vi "E517_Simple_Test.vi"(0 "System no.":i32=1 min=1 step=1, 5 "error in":errorcluster, 6 "Interface":u16(ring) items=["RS232", "GPIB", "TCP/IP", "USB"], 7 "Timeout":u32=5000, 8 "RS232 settings":cluster{"Portnumber":i32, "Baudrate":u16}={"Portnumber"=0, "Baudrate"=5} {"Portnumber" items=["COM1", "COM2", "COM3", "COM4", "COM5", "COM6", "COM7", "COM8", "COM9", "COM10", "COM11", "COM12", "COM13", "COM14", "COM15", "COM16", "COM17", "COM18", "COM19", "COM20", "COM21", "COM22", "COM23", "COM24", "COM25", "COM26", "COM27", "COM28", "COM29", "COM30"]; "Baudrate" items=["9600", "14400", "19200", "38400", "57600", "115200"]}, 9 "GPIB settings":cluster{"Bus":i32, "Address":i32}={"Bus"=0, "Address"=4}, 10 "TCP/IP settings":T1={"Host address/name"="localhost", "Port"=50000, "Board"=0, "TCP/IP Search?"=TRUE}, 11 "USB settings":cluster{"S/N":string, "USB Search?":bool}={"S/N"="", "USB Search?"=TRUE}) -> (14 "Identification":string, 15 "Helpstring":string, 16 "Axis IDs":string[](array[string]), 17 "Position":dbl[](array[numeric]) format="%.6f", 19 "error out":errorcluster)   [LabVIEW 2011]
doc: "This simple test VI is a stand-alone sample application. Use the \nHelp - Show Context Help menu sequence in the LabVIEW environment to display the Context Help window with the VI and control/indicator descriptions.\n\nSpecify \n¢ System no. (= 1 in a one-system configuration),\n¢ Interface (= RS232, GPIB, TCP/IP or USB)\n¢ Timeout value (in milliseconds)\n¢ and interface settings first.\n\nThen start the VI. The VI will open a connection to the E-517 and query the controller for its identification string (*IDN?), help string (HLP?), the IDs (SAI?) and their current position values (POS?). The diagram shows how to combine the driver and support VIs for these tasks."
panel:
  # "Simple E-517 communication test program"
  # "Select E-517 interface, timeout value and interface settings first, then start the VI. The VI will open the chosen port, query for the available axis IDs \n(SAI?), position (POS?), identification (*IDN?) and the help string (HLP?). See VI and control/ indicator information for details."
  # "Only for\nInterface = RS232:"
  # "Only for\nInterface = GPIB:"
  # "Only for Interface = USB:"
  # "Only for Interface =  TCP/IP:"
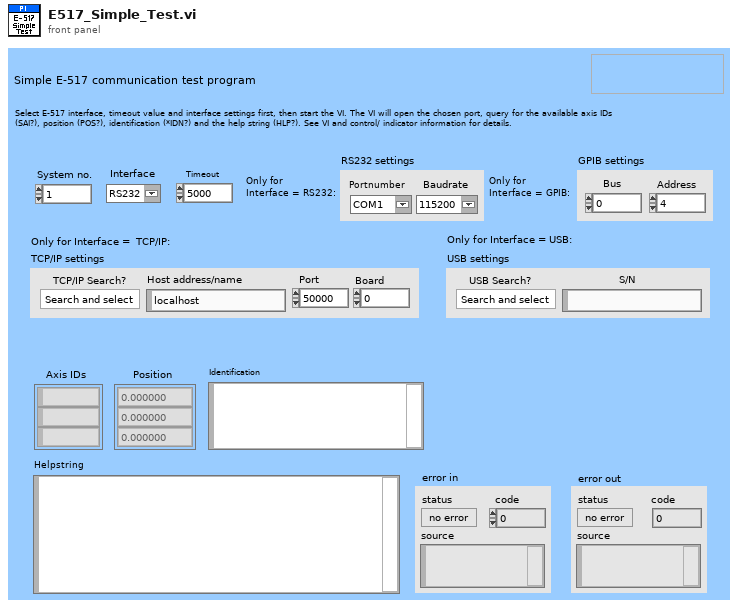
[diagram p1: front panel]
types:
  T1 = cluster{"Host address/name":string, "Port":i32, "Board":i32, "TCP/IP Search?":bool}
  T2 = cluster{"Host address/name":string, "Port":i32, "Board":i32}
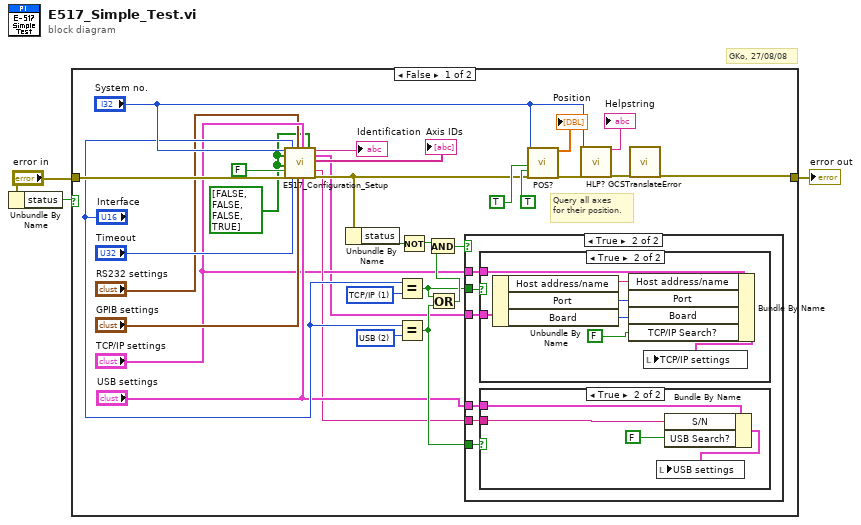
[diagram p0: block diagram]
diagram:
  # "GKo, 27/08/08"
  n1 = Unbundle By Name("error in") -> ("status"=w1:bool)
  n2 = case shown="False" w1 {
    tunnel: [w27 w51] -> w2
    tunnel: "error in" -> [w25 w51]
    frame False {
      w4 = bool[] [FALSE, FALSE, FALSE, TRUE] ("Axes to set online")
      w16 = u16 2 items=["RS232", "TCP/IP", "USB"] ("Interface")
      w17 = u16 1 items=["RS232", "TCP/IP", "USB"] ("Interface")
      # "Query all axes\nfor their position."
      n3 = call "E517_Configuration_Setup.vi"("System no."="System no.", "Set channel online?"=w4, "Switch servo on?"=w4, "Stop wave generator\noutput (if any)"=FALSE ("Stop wave generator\noutput (if any)"), "error in"=w25, "Interface"="Interface", "Timeout"="Timeout", "RS232 settings"="RS232 settings", "GPIB settings"="GPIB settings", "TCP/IP settings"="TCP/IP settings", "USB settings"="USB settings", "Axes to move to middle"=w4) -> ("Identification"=→"Identification":string, "TCP/IP settings out"=w7:T2, "Conn. Axes"=→"Axis IDs":string[], "USB: S/N out"=w9:string, "error out"=w12:errorcluster)  [unwired: 1 in, 2 out]
      n4 = Unbundle By Name(w12) -> ("status"=w20:bool)
      n5 = Equal?(x="Interface", y=w17) -> (x = y?=w14:bool)
      n6 = Equal?(x="Interface", y=w16) -> (x = y?=w13:bool)
      n7 = Not(x=w20) -> (.not. x?=w18:bool)
      n8 = Or(x=w14, y=w13) -> (x .or. y?=w15:bool)
      n9 = And(x=w18, y=w15) -> (x .and. y?=w19:bool)
      n10 = case shown="True" w19 {
        tunnel: "TCP/IP settings" -> [_ w39]
        tunnel: w7 -> [_ w38]
        tunnel: w9 -> [_ w36]
        tunnel: "USB settings" -> [_ w37]
        tunnel: w14 -> [_ w35]
        tunnel: w13 -> [_ w34]
        frame False {
        }
        frame True {
          n11 = case shown="True" w35 {
            tunnel: w39 -> [_ w49]
            tunnel: w38 -> [_ w47]
            frame False {
            }
            frame True {
              n12 = Unbundle By Name(w47) -> ("Host address/name"=w46:string, "Port"=w45:i32, "Board"=w44:i32)
              n13 = Bundle By Name(cluster=w49, "Host address/name"=w46, "Port"=w45, "Board"=w44, "TCP/IP Search?"=FALSE) -> (w50:T1)
              n14 = local write "TCP/IP settings"(w50) -> ()
            }
          }
          n15 = case shown="True" w34 {
            tunnel: w37 -> [_ w43]
            tunnel: w36 -> [_ w41]
            frame False {
            }
            frame True {
              n16 = Bundle By Name(cluster=w43, "S/N"=w41, "USB Search?"=FALSE ("TCP/IP Search?")) -> (w40:cluster{"S/N":string, "USB Search?":bool})
              n17 = local write "USB settings"(w40) -> ()
            }
          }
        }
      }
      n18 = call "POS?.vi"("System no."="System no.", "All axes?"=TRUE, "Axis identifier?"=TRUE, "error in"=w12) -> ("Position"=→"Position":dbl[], "error out"=w31:errorcluster)  [unwired: 1 in, 13 out]
      n19 = call "HLP?.vi"("System no."="System no.", "error in"=w31) -> ("Help string"=→"Helpstring":string, "error out"=w28:errorcluster)  [unwired: 16 out]
      n20 = call "GCSTranslateError.vi"("error in"=w28) -> ("error out"=w27:errorcluster)  [unwired: 18 out]
    }
    frame True {
    }
  }
  "error out" <- w2
